vi "Minify.vi"(4 "Disable LabVIEW Extensions":bool, 8 "error in (no error)":errorcluster, 10 "Offset":i32, 11 "JSON":string) -> (0 "error out":errorcluster, 2 "Rest of Input String":string, 3 "<JSON>":string caption="<JSON>First JSON Value")   [LabVIEW 2020, in "JSONtext.lvlib"]
doc: "\"Minify\" a JSON Value, removing all whitespace (and stripping any comments)."
uses:
  <vilib>/JDP Science/JSONtext/JSONtext.lvlib
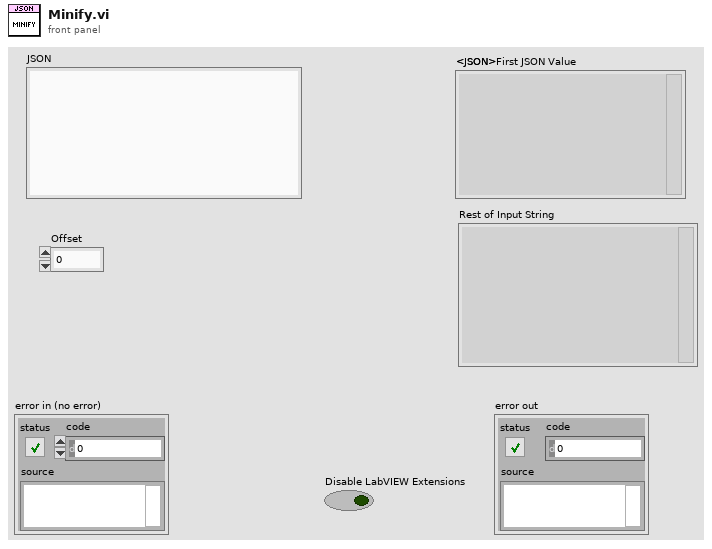
[diagram p1: front panel]
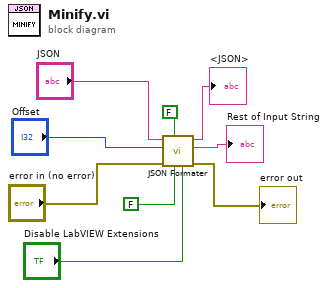
[diagram p0: block diagram]
diagram:
  n1 = call <vilib>:"JSON Formater.vi"("Disable LabVIEW Extensions"="Disable LabVIEW Extensions", "Pretty Print"=FALSE, "Comment out unparsable lines"=FALSE ("Convert Unparsable lines into Comments"), "error in"="error in (no error)", "Offset"="Offset", "JSON"="JSON") -> ("error OUT"=→"error out":errorcluster, "Rest of Input String"=→"Rest of Input String":string, "<JSON>"=→"<JSON>":string)  [unwired: 3 in]
